vi "vertcat.vi"(8 "error in (no error)":errorcluster, 9 "A1":dbl[][](array[numeric]), 11 "A0":dbl[][](array[numeric])) -> (0 "error out":errorcluster, 3 "Stacked 2D Array":dbl[][](array[numeric]))   [LabVIEW 2016]
doc: "Vertical concatenate 2D arrays of A0 and A1. New 2D array is [A0; A1]."
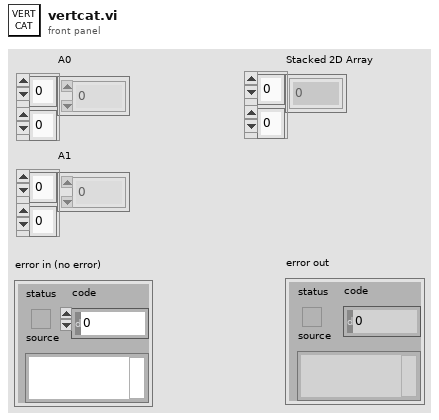
[diagram p1: front panel]
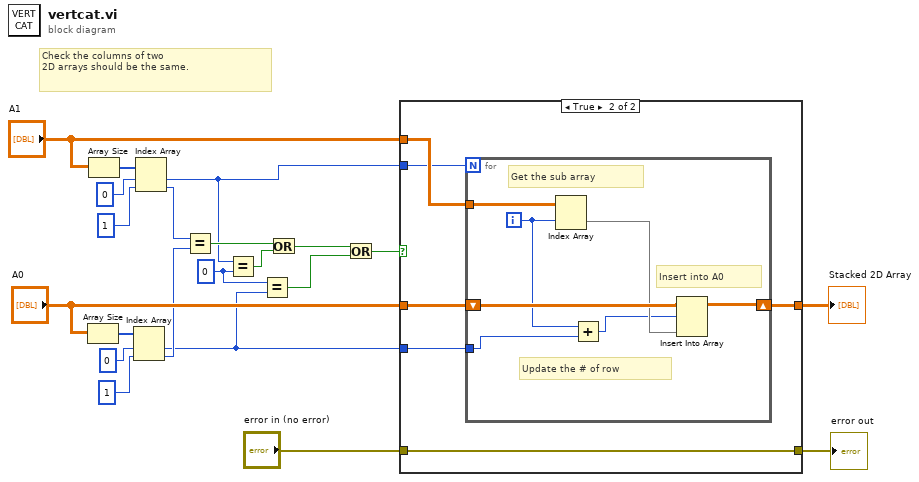
[diagram p0: block diagram]
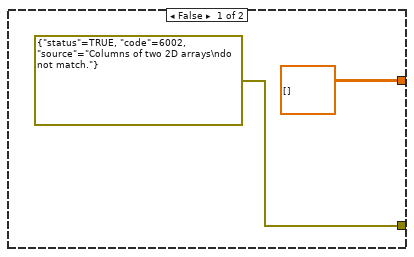
[diagram p2: hidden frame]
diagram:
  w2 = 0 ("y")
  # "Check the columns of two\n2D arrays should be the same."
  n1 = Array Size(array="A0") -> (size(s)=w17:i32[])
  n2 = Array Size(array="A1") -> (size(s)=w18:i32[])
  n3 = Index Array(array=w17, index #1=0 ("index"), index #2=1 ("index")) -> (element #1=w1:i32, element #2=w9:i32)
  n4 = Index Array(array=w18, index #1=0 ("index"), index #2=1 ("index")) -> (element #1=w6:i32, element #2=w13:i32)
  n5 = Equal?(x=w13, y=w9) -> (x = y?=w8:bool)
  n6 = Equal?(x=w6, y=w2) -> (x = y?=w7:bool)
  n7 = Equal?(x=w2, y=w1) -> (x = y?=w4:bool)
  n8 = Or(x=w8, y=w7) -> (x .or. y?=w5:bool)
  n9 = Or(x=w5, y=w4) -> (x .or. y?=w3:bool)
  n10 = case shown="True" w3 {
    tunnel: [dbl[][] [] ("A0") w29] -> w21
    tunnel: "A1" -> [_ w28]
    tunnel: "A0" -> [_ w27]
    tunnel: "error in (no error)" -> [_ w26]
    tunnel: [errorcluster {"status"=TRUE, "code"=6002, "source"="Columns of two 2D arrays\ndo not match."} ("error in (no error)") w26] -> w15
    tunnel: w6 -> [_ w25]
    tunnel: w1 -> [_ w24]
    frame False {
    }
    frame True {
      n11 = for {
        N: w25 -> [_]
        shift-right: [w33] -> w29
        shift-left: w27 -> [w35]
        tunnel: w28 -> [w36]
        tunnel: w24 -> [w30]
        i -> [w31]
        # "Insert into A0"
        # "Get the sub array"
        # "Update the # of row"
        n12 = Index Array(array=w36, index (row)=w31) -> (element=w34:dbl[])  [unwired: 1 in]
        n13 = Add(x=w31, y=w30) -> (x+y=w32:i32)
        n14 = Insert Into Array(array=w35, index (row)=w32, new element=w34) -> (w33:dbl[][])  [unwired: 1 in]
      }
    }
  }
  "Stacked 2D Array" <- w21
  "error out" <- w15
